vi "PopupWindow.vi"() -> ()   [LabVIEW 2012]
uses:
  <resource>/importtools/Common/Event/NISAST Event.lvclass
panel:
  out "数据字符串":string
  out "类型字符串":i16[](array[numeric])
  in  "Event In":refnum<class "NISAST Event.lvclass">
  in  "取消按钮":bool
  in  "确定按钮":bool
  out "布尔":bool
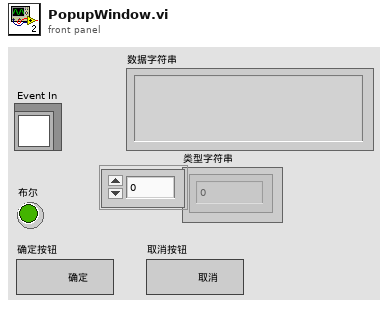
[diagram p1: front panel]
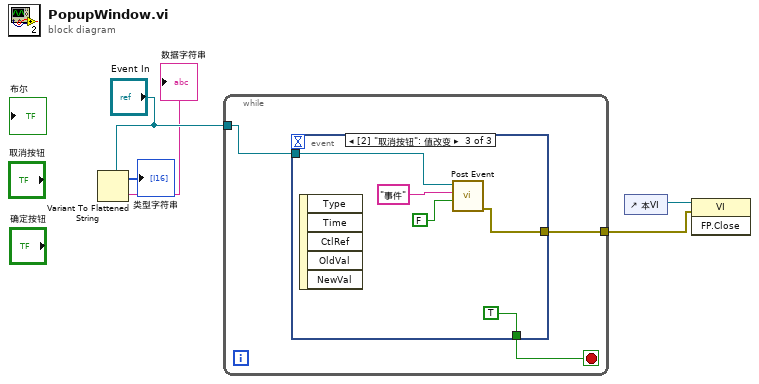
[diagram p0: block diagram]
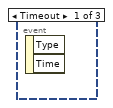
[diagram p2: hidden frame]
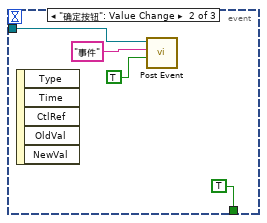
[diagram p3: hidden frame]
diagram:
  n1 = Variant To Flattened String(Variant="Event In") -> (data string=→"数据字符串":string, 1:→"类型字符串":i16[])
  n2 = while {
    tunnel: "Event In" -> [w7]
    tunnel: [w6] -> w4
    stop <- w8 stop-if-true
    n3 = event shown="[2] \"取消按钮\": 值改变" {
      selector: _ -> [_ _ _]
      dyn-events: _ -> [_ _ _]
      timeout: _ -> [_ _ _]
      tunnel: [_ TRUE TRUE] -> w8
      tunnel: w7 -> [_ w11 w14]
      tunnel: [_ _ w13] -> w6
      event Timeout {
        n4 = event-data() -> ()  [unwired: 1 in, 2 out]
      }
      event "确定按钮": Value Change {
        n5 = event-data() -> ()  [unwired: 1 in, 5 out]
        n6 = call-dynamic "Post Event.vi"("Event Data"=TRUE, "Event Name"="事件", "Event in"=w11) -> ()  [unwired: 7 in, 2 out]
      }
      event "取消按钮": Value Change {
        n7 = event-data() -> ()  [unwired: 1 in, 5 out]
        n8 = call-dynamic "Post Event.vi"("Event Data"=FALSE, "Event Name"="事件", "Event in"=w14) -> ("error out"=w13:errorcluster)  [unwired: 7 in, 1 out]
      }
    }
  }
  n9 = control-ref of="本VI"() -> (w5:refnum<vi>)
  n10 = invoke class="VI" method="FP.Close"(reference=w5, error in=w4) -> ()  [unwired: 1 in, 3 out]
